vi "UDP Sender.vi"() -> ()   [LabVIEW 2010]
doc: "This VI is designed to be used with the UDP Receiver VI. Run the UDP Receiver.vi first.\n\nThe UDP protocol differs from TCP in that there is no error-checking with the packets of information that are sent, and thus no guarantee whatsoever that an intended recipient will actually receive a given piece of data.\n\nUDP does offer the ability to \"broadcast\" data across a network--simply specify an IP Address of all ones (255.255.255.255) to attempt to broadcast information network-wide. Keep in mind that routers and other network hardware will generally refuse to forward the broadcast beyond certain points, so the extent of the broadcast will in practice be limited."
panel:
  in  "# Repetitions":i32=10
  in  "Remote Port":u16=61557
  in  "Local Port":u16=61556
  in  "Remote Host":string="localhost"
  in  "Data String":string="<data>"
  in  "broadcast":bool
  # "Instructions:\n1. Open the UDP Receiver.vi located in the same library.\n2. Make sure that the Remote Port in this VI and the Port in the UDP Receive.vi are the same.\n3. Press the button if you want to broadcast the data to all the network, instead of sending it to a specific address.\n4. Change the number of times you want to send the data to the receiver in the # of Repetitions control.\n5. Follow the instructions on it's front panel.\nNote: This VI is built to work with the UDP Receiver.vi."
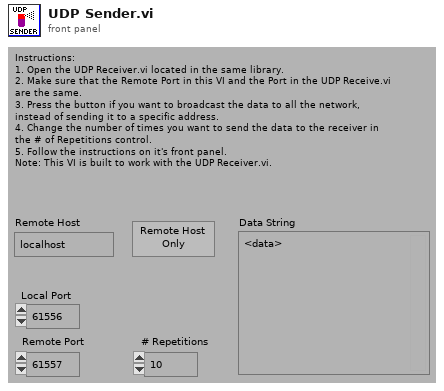
[diagram p1: front panel]
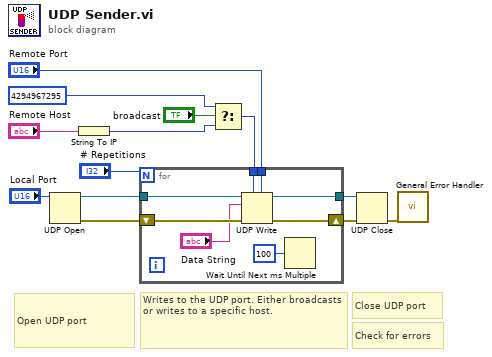
[diagram p0: block diagram]
diagram:
  # "Close UDP port"
  # "Check for errors"
  # "Writes to the UDP port. Either broadcasts or writes to a specific host."
  # "Open UDP port"
  n1 = UDP Open(11:"Local Port") -> (port=w13:refnum<k16>, 0:w11:errorcluster)  [unwired: 1 in, 4 out]
  n2 = String To IP(1:"Remote Host") -> (0:w5:u32)
  n3 = Select(t=u32 4294967295, s="broadcast", f=w5) -> (s? t:f=w4:u32)
  n4 = for {
    N: "# Repetitions" -> [_]
    tunnel: w13 -> [w19]
    tunnel: w4 -> [w21]
    tunnel: "Remote Port" -> [w20]
    shift-right: [w17] -> w10
    shift-left: w11 -> [w18]
    tunnel: [w16] -> w9
    n5 = UDP Write(address=w21, port or service name=w20, connection ID=w19, data in="Data String", 8:w18) -> (error out=w17:errorcluster, 3:w16:refnum<k16>)  [unwired: 1 out]
    n6 = Wait Until Next ms Multiple(millisecond multiple=u32 100) -> ()  [unwired: 1 out]
  }
  n7 = UDP Close(connection ID=w9, 8:w10) -> (error out=w8:errorcluster)  [unwired: 1 out]
  n8 = call <vilib>:"General Error Handler.vi"("error in (no error)"=w8) -> ()  [unwired: 1 in, 14 out]
